vi "nana_4-solanka.vi"() -> ()   [LabVIEW 2015]
uses:
  <vilib>/MakerHub/LINX/Public/Peripherals/Digital/Digital Write N Chans.vi
  <vilib>/MakerHub/LINX/Public/Peripherals/Analog/Analog Read 1 Chan.vi
  <vilib>/MakerHub/LINX/Private/Local IO/LinxDigitalWrite.vi
  <vilib>/MakerHub/LINX/Public/Utilities/Check Channel.vi
  <vilib>/MakerHub/LINX/Public/Peripherals/Analog/Analog Read N Chans.vi
  <vilib>/MakerHub/LINX/Private/Local IO/LinxAnalogRead.vi
  <vilib>/MakerHub/LINX/Public/Utilities/Open Serial.vi
  <vilib>/MakerHub/LINX/Private/Utilties/Generate Error.vi
  <vilib>/MakerHub/LINX/LMH-LINX.lvlib
panel:
  in  "time post":u32
  in  "number of pulses":i32
  in  "low delay":u32
  in  "peak delay":u32
  out "Ref":dbl(graph)
  in  "LED":refnum<visa-resource-name>="N/A"
  out "3":dbl(graph)
  out "2":dbl(graph)
  out "4":dbl(graph)
  out "1":dbl(graph)
  out "pos":dbl
  in  "milliseconds to wait":u32
  in  "time pre":u32
  in  "Serial Port Analog":refnum<visa-resource-name>="N/A"
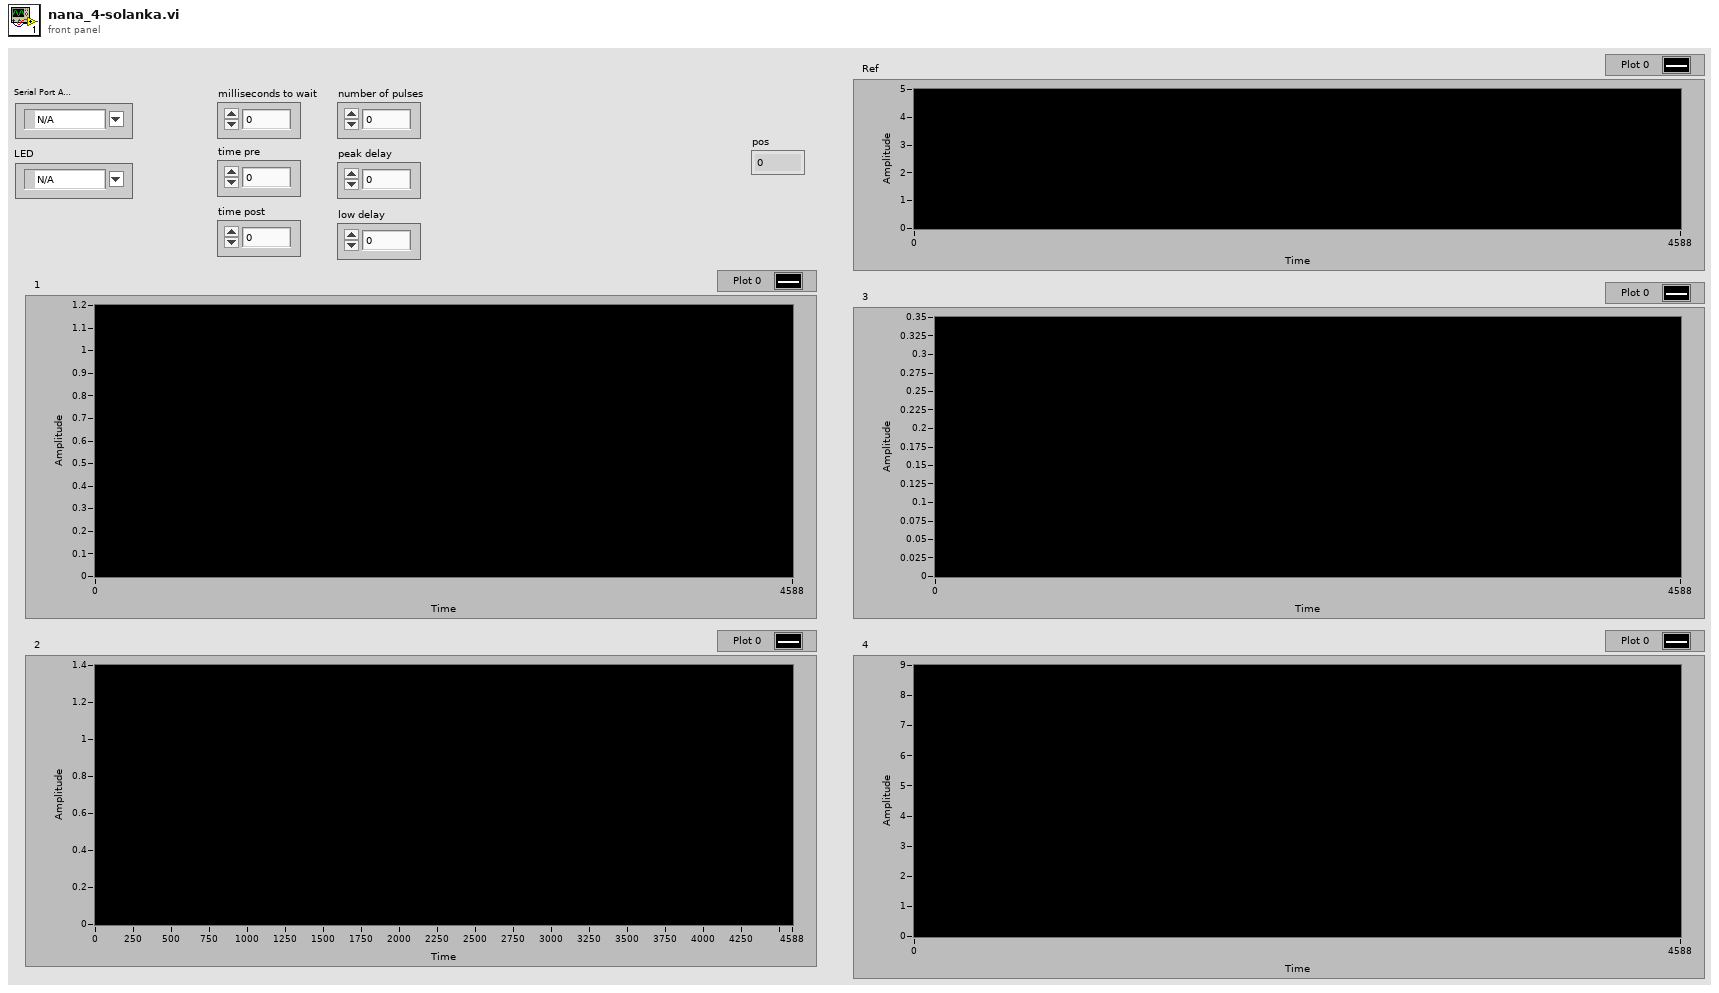
[diagram p1: front panel]
types:
  T1 = typedef "LMH-LINX.lvlib/LINX Ref.ctl" = cluster{"IO":T2, "Interface":T3, "LINX Device Config":T4}
  T2 = typedef "LMH-LINX.lvlib/Platform.ctl" = enum16{"Remote", "Local"}
  T3 = typedef "LMH-LINX.lvlib/Interface.ctl" = enum16{"Serial", "TCP"}
  T4 = typedef "LMH-LINX.lvlib/Device.lvlib/LINX Device Config.ctl" = cluster{"Interface":T3, "COM Port":refnum<visa-resource-name>, "TCP Configuration":T5, "Device Family":u8, "Device ID":u8, "Device Name":string, "TCP Ref":refnum<k5>, "Channels":T6}
  T5 = typedef "LMH-LINX.lvlib/Device.lvlib/TCP Config.ctl" = cluster{"IP Address":string, "Port":u16}
  T6 = typedef "LMH-LINX.lvlib/Channels.ctl" = cluster{"DI":u8[], "DO":u8[], "AI":u8[], "AO":u8[], "PWM":u8[], "QE":u8[], "UART":u8[], "I2C 2":u8[], "SPI":u8[], "CAN":u8[], "Servo":u8[], "AI Ref (V)":dbl, "AI Resolution (Bits)":u8, "AO Ref (V)":dbl, "AO Resolution (Bits)":u8}
  T7 = enum16{"open", "replace", "create", "open or create", "replace or create", "replace or create with confirmation"}
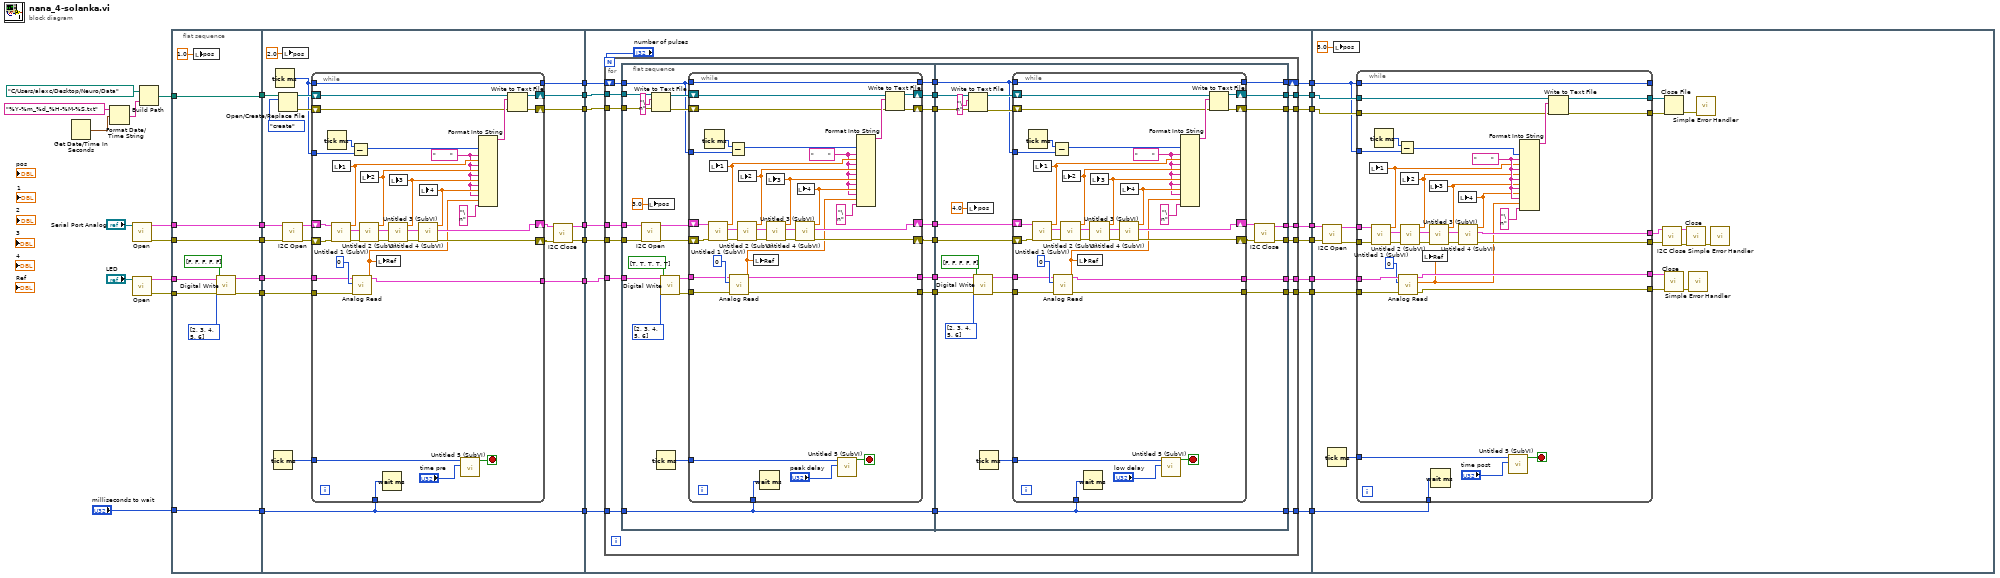
[diagram p0: block diagram]
diagram:
  n1 = Get Date/Time In Seconds() -> (seconds since 1Jan1904=w11:timestamp)
  n2 = Format Date/Time String(time format string (%c)="%Y-%m_%d_%H-%M-%S.txt", seconds (now)=w11) -> (date/time string=w13:string)  [unwired: 1 in]
  n3 = call-poly <vilib>:"Open.vi"("Serial Port"="Serial Port Analog") -> ("Error Out"=w17:errorcluster, "LINX Resource"=w18:T1)  [unwired: 8 in, 1 out]
  n4 = call-poly <vilib>:"Open.vi"("Serial Port"="LED") -> ("Error Out"=w8:errorcluster, "LINX Resource"=w9:T1)  [unwired: 8 in, 1 out]
  n5 = Build Path(base path=path "C:/Users/alexc/Desktop/Neuro/Data", name or relative path=w13) -> (appended path=w10:path)
  n6 = flat-sequence {
    tunnel: [w41] -> w33
    tunnel: [w40] -> w32
    tunnel: [w39] -> w29
    tunnel: [w34] -> w20
    tunnel: w18 -> [w41]
    tunnel: w17 -> [w40]
    tunnel: w10 -> [w39]
    tunnel: w9 -> [w38]
    tunnel: w8 -> [w37]
    tunnel: [w36] -> w7
    tunnel: [w35] -> w6
    tunnel: "milliseconds to wait" -> [w34]
    tunnel: w33 -> [w66]
    tunnel: w32 -> [w65]
    tunnel: [w64] -> w31
    tunnel: [w63] -> w30
    tunnel: w29 -> [w62]
    tunnel: [w58] -> w28
    tunnel: [w57] -> w27
    tunnel: [w55] -> w26
    tunnel: w20 -> [w53]
    tunnel: [w53] -> w19
    tunnel: w7 -> [w47]
    tunnel: w6 -> [w46]
    tunnel: [w45] -> w5
    tunnel: [w105] -> w25
    tunnel: [w104] -> w24
    tunnel: [w108] -> w23
    tunnel: [w107] -> w22
    tunnel: [w106] -> w21
    tunnel: w19 -> [w109]
    tunnel: w26 -> [w113]
    tunnel: w27 -> [w114]
    tunnel: w28 -> [w115]
    tunnel: w30 -> [w111]
    tunnel: w31 -> [w112]
    tunnel: w5 -> [w116]
    tunnel: [w103] -> w3
    tunnel: [w102] -> w2
    tunnel: [w101] -> w1
    tunnel: w21 -> [w274]
    tunnel: w22 -> [w275]
    tunnel: w23 -> [w261]
    tunnel: w24 -> [w279]
    tunnel: w25 -> [w283]
    tunnel: w3 -> [w278]
    tunnel: w2 -> [w265]
    tunnel: w1 -> [w264]
    frame #0 {
      n7 = local write "pos"(1.0 ("pos")) -> ()
      n8 = call-poly <vilib>:"Digital Write.vi"("Error In"=w37, "Values"=bool[] [FALSE, FALSE, FALSE, FALSE, FALSE], "DO Channels"=u8[] [2, 3, 4, 5, 6], "LINX Resource"=w38) -> ("Error Out"=w35:errorcluster, "LINX Resource"=w36:T1)  [unwired: 6 in]
    }
    frame #1 {
      n9 = Tick Count (ms)() -> (millisecond timer value=w54:u32)
      n10 = Tick Count (ms)() -> (millisecond timer value=w56:u32)
      n11 = Open/Create/Replace File(file path (use dialog)=w62, operation (0:open)=T7."create") -> (refnum out=w60:refnum<file>, error out=w59:errorcluster)  [unwired: 4 in, 1 out]
      n12 = local write "pos"(2.0 ("pos")) -> ()
      n13 = call <vilib>:"I2C Open.vi"("Error In"=w65, "LINX Resource"=w66) -> ("Error Out"=w51:errorcluster, "LINX Resource"=w52:T1)  [unwired: 8 in]
      n14 = while {
        tunnel: w56 -> [w93]
        shift-right: [w89] -> w58
        shift-left: w60 -> [w91]
        shift-right: [w88] -> w57
        shift-left: w59 -> [w90]
        tunnel: [w87] -> w55
        tunnel: w56 -> [w87]
        tunnel: w54 -> [w86]
        tunnel: w53 -> [w68]
        shift-right: [w83] -> w50
        shift-left: w52 -> [w85]
        shift-right: [w82] -> w49
        shift-left: w51 -> [w84]
        tunnel: w47 -> [w71]
        tunnel: w46 -> [w70]
        tunnel: [w67] -> w45
        stop <- w69 stop-if-true
        w75 = "       "
        n15 = Tick Count (ms)() -> (millisecond timer value=w94:u32)
        n16 = call "Untitled 1 (SubVI).vi"("error in (no error)"=w84, "LINX Resource in"=w85) -> ("error out"=w99:errorcluster, "LINX Resource out"=w100:T1, "Numeric"=w80:dbl)  [unwired: 7 in]
        n17 = local write "1"(w80) -> ()
        n18 = Subtract(x=w94, y=w93) -> (x-y=w76:u32)
        n19 = call-poly <vilib>:"Analog Read.vi"("Error In"=w70, "Analog Channel"=u8 0, "LINX Resource"=w71) -> ("Voltage"=w72:dbl, "LINX Resource"=w67:T1)  [unwired: 5 in, 2 out]
        n20 = call "Untitled 2 (SubVI).vi"("error in (no error)"=w99, "LINX Resource in"=w100) -> ("error out"=w98:errorcluster, "LINX Resource"=w97:T1, "Numeric"=w79:dbl)  [unwired: 7 in]
        n21 = local write "2"(w79) -> ()
        n22 = local write "Ref"(w72) -> ()
        n23 = Wait (ms)(milliseconds to wait=w68) -> ()  [unwired: 1 out]
        n24 = call "Untitled 3 (SubVI).vi"("error in (no error)"=w98, "LINX Resource in"=w97) -> ("error out"=w95:errorcluster, "LINX Resource out"=w96:T1, "Numeric"=w78:dbl)  [unwired: 7 in]
        n25 = local write "3"(w78) -> ()
        n26 = call "Untitled 4 (SubVI).vi"("error in (no error)"=w95, "LINX Resource in"=w96) -> ("error out"=w82:errorcluster, "LINX Resource"=w83:T1, "Numeric"=w81:dbl)  [unwired: 7 in]
        n27 = local write "4"(w81) -> ()
        n28 = call "Untitled 5 (SubVI).vi"("time_1"="time pre", "millisecond timer value"=w86) -> ("Boolean"=w69:bool)  [unwired: 9 in]
        n29 = Format Into String(w76, w75, w80, w75, w79, w75, w78, w75, w81, w75, w72, "\n") -> (resulting string=w92:string)  [unwired: 3 in, 1 out]
        n30 = Write to Text File(file (use dialog)=w91, text=w92, error in=w90) -> (refnum out=w89:refnum<file>, error out=w88:errorcluster)  [unwired: 1 in, 1 out]
      }
      n31 = call <vilib>:"I2C Close.vi"("Error In"=w49, "LINX Resource"=w50) -> ("Error Out"=w63:errorcluster, "LINX Resource"=w64:T1)  [unwired: 8 in]
    }
    frame #2 {
      n32 = for {
        N: "number of pulses" -> [_]
        tunnel: w116 -> [w139]
        tunnel: w115 -> [w138]
        tunnel: w114 -> [w137]
        shift-right: [w124] -> w108
        shift-left: w113 -> [w134]
        tunnel: w112 -> [w136]
        tunnel: w111 -> [w135]
        tunnel: w109 -> [w126]
        tunnel: [w123] -> w107
        tunnel: [w122] -> w106
        tunnel: [w121] -> w105
        tunnel: [w120] -> w104
        tunnel: [w119] -> w103
        tunnel: [w118] -> w102
        tunnel: [w117] -> w101
        n33 = flat-sequence {
          tunnel: w139 -> [w159]
          tunnel: w138 -> [w156]
          tunnel: w137 -> [w155]
          tunnel: w136 -> [w148]
          tunnel: w135 -> [w147]
          tunnel: w134 -> [w144]
          tunnel: [w163] -> w133
          tunnel: [w162] -> w132
          tunnel: [w158] -> w131
          tunnel: [w157] -> w130
          tunnel: [w152] -> w129
          tunnel: [w151] -> w128
          tunnel: [w143] -> w127
          tunnel: w126 -> [w140]
          tunnel: [w140] -> w125
          tunnel: w133 -> [w218]
          tunnel: w132 -> [w217]
          tunnel: w131 -> [w212]
          tunnel: w130 -> [w211]
          tunnel: w129 -> [w214]
          tunnel: w128 -> [w213]
          tunnel: w127 -> [w210]
          tunnel: w125 -> [w202]
          tunnel: [w207] -> w124
          tunnel: [w206] -> w123
          tunnel: [w205] -> w122
          tunnel: [w204] -> w121
          tunnel: [w203] -> w120
          tunnel: [w202] -> w119
          tunnel: [w201] -> w118
          tunnel: [w200] -> w117
          frame #0 {
            n34 = call <vilib>:"I2C Open.vi"("Error In"=w147, "LINX Resource"=w148) -> ("Error Out"=w145:errorcluster, "LINX Resource"=w146:T1)  [unwired: 8 in]
            n35 = local write "pos"(3.0 ("pos")) -> ()
            n36 = Write to Text File(file (use dialog)=w156, text="\n", error in=w155) -> (refnum out=w154:refnum<file>, error out=w153:errorcluster)  [unwired: 1 in, 1 out]
            n37 = Tick Count (ms)() -> (millisecond timer value=w141:u32)
            n38 = call-poly <vilib>:"Digital Write.vi"("Values"=bool[] [TRUE, TRUE, TRUE, TRUE, TRUE], "DO Channels"=u8[] [2, 3, 4, 5, 6], "LINX Resource"=w159) -> ("Error Out"=w150:errorcluster, "LINX Resource"=w149:T1)  [unwired: 7 in]
            n39 = while {
              tunnel: w144 -> [w192]
              shift-right: [w188] -> w158
              shift-left: w154 -> [w190]
              shift-right: [w187] -> w157
              shift-left: w153 -> [w189]
              tunnel: [w186] -> w143
              tunnel: w144 -> [w186]
              tunnel: w141 -> [w185]
              tunnel: w140 -> [w167]
              shift-right: [w182] -> w163
              shift-left: w146 -> [w184]
              shift-right: [w181] -> w162
              shift-left: w145 -> [w183]
              tunnel: w149 -> [w170]
              tunnel: w150 -> [w169]
              tunnel: [w166] -> w152
              tunnel: [w165] -> w151
              stop <- w168 stop-if-true
              w174 = "       "
              n40 = Tick Count (ms)() -> (millisecond timer value=w193:u32)
              n41 = call "Untitled 1 (SubVI).vi"("error in (no error)"=w183, "LINX Resource in"=w184) -> ("error out"=w198:errorcluster, "LINX Resource out"=w199:T1, "Numeric"=w179:dbl)  [unwired: 7 in]
              n42 = local write "1"(w179) -> ()
              n43 = Subtract(x=w193, y=w192) -> (x-y=w175:u32)
              n44 = call-poly <vilib>:"Analog Read.vi"("Error In"=w169, "Analog Channel"=u8 0, "LINX Resource"=w170) -> ("Error Out"=w165:errorcluster, "Voltage"=w171:dbl, "LINX Resource"=w166:T1)  [unwired: 5 in, 1 out]
              n45 = call "Untitled 2 (SubVI).vi"("error in (no error)"=w198, "LINX Resource in"=w199) -> ("error out"=w197:errorcluster, "LINX Resource"=w196:T1, "Numeric"=w178:dbl)  [unwired: 7 in]
              n46 = local write "2"(w178) -> ()
              n47 = local write "Ref"(w171) -> ()
              n48 = Wait (ms)(milliseconds to wait=w167) -> ()  [unwired: 1 out]
              n49 = call "Untitled 3 (SubVI).vi"("error in (no error)"=w197, "LINX Resource in"=w196) -> ("error out"=w194:errorcluster, "LINX Resource out"=w195:T1, "Numeric"=w177:dbl)  [unwired: 7 in]
              n50 = local write "3"(w177) -> ()
              n51 = call "Untitled 4 (SubVI).vi"("error in (no error)"=w194, "LINX Resource in"=w195) -> ("error out"=w181:errorcluster, "LINX Resource"=w182:T1, "Numeric"=w180:dbl)  [unwired: 7 in]
              n52 = local write "4"(w180) -> ()
              n53 = call "Untitled 5 (SubVI).vi"("time_1"="peak delay", "millisecond timer value"=w185) -> ("Boolean"=w168:bool)  [unwired: 9 in]
              n54 = Format Into String(w175, w174, w179, w174, w178, w174, w177, w174, w180, w174, w171, "\n") -> (resulting string=w191:string)  [unwired: 3 in, 1 out]
              n55 = Write to Text File(file (use dialog)=w190, text=w191, error in=w189) -> (refnum out=w188:refnum<file>, error out=w187:errorcluster)  [unwired: 1 in, 1 out]
            }
          }
          frame #1 {
            n56 = local write "pos"(4.0 ("pos")) -> ()
            n57 = Write to Text File(file (use dialog)=w212, text="\n", error in=w211) -> (refnum out=w220:refnum<file>, error out=w221:errorcluster)  [unwired: 1 in, 1 out]
            n58 = call-poly <vilib>:"Digital Write.vi"("Error In"=w213, "Values"=bool[] [FALSE, FALSE, FALSE, FALSE, FALSE], "DO Channels"=u8[] [2, 3, 4, 5, 6], "LINX Resource"=w214) -> ("Error Out"=w225:errorcluster, "LINX Resource"=w224:T1)  [unwired: 6 in]
            n59 = Tick Count (ms)() -> (millisecond timer value=w208:u32)
            n60 = while {
              tunnel: w210 -> [w253]
              shift-right: [w249] -> w206
              shift-left: w220 -> [w251]
              shift-right: [w248] -> w205
              shift-left: w221 -> [w250]
              tunnel: [w247] -> w207
              tunnel: w210 -> [w247]
              tunnel: w208 -> [w246]
              tunnel: w202 -> [w228]
              shift-right: [w243] -> w216
              shift-left: w218 -> [w245]
              shift-right: [w242] -> w215
              shift-left: w217 -> [w244]
              tunnel: w224 -> [w231]
              tunnel: w225 -> [w230]
              tunnel: [w227] -> w201
              tunnel: [w226] -> w200
              stop <- w229 stop-if-true
              w235 = "       "
              n61 = Tick Count (ms)() -> (millisecond timer value=w254:u32)
              n62 = call "Untitled 1 (SubVI).vi"("error in (no error)"=w244, "LINX Resource in"=w245) -> ("error out"=w259:errorcluster, "LINX Resource out"=w260:T1, "Numeric"=w240:dbl)  [unwired: 7 in]
              n63 = local write "1"(w240) -> ()
              n64 = Subtract(x=w254, y=w253) -> (x-y=w236:u32)
              n65 = call-poly <vilib>:"Analog Read.vi"("Error In"=w230, "Analog Channel"=u8 0, "LINX Resource"=w231) -> ("Error Out"=w226:errorcluster, "Voltage"=w232:dbl, "LINX Resource"=w227:T1)  [unwired: 5 in, 1 out]
              n66 = call "Untitled 2 (SubVI).vi"("error in (no error)"=w259, "LINX Resource in"=w260) -> ("error out"=w258:errorcluster, "LINX Resource"=w257:T1, "Numeric"=w239:dbl)  [unwired: 7 in]
              n67 = local write "2"(w239) -> ()
              n68 = local write "Ref"(w232) -> ()
              n69 = Wait (ms)(milliseconds to wait=w228) -> ()  [unwired: 1 out]
              n70 = call "Untitled 3 (SubVI).vi"("error in (no error)"=w258, "LINX Resource in"=w257) -> ("error out"=w255:errorcluster, "LINX Resource out"=w256:T1, "Numeric"=w238:dbl)  [unwired: 7 in]
              n71 = local write "3"(w238) -> ()
              n72 = call "Untitled 4 (SubVI).vi"("error in (no error)"=w255, "LINX Resource in"=w256) -> ("error out"=w242:errorcluster, "LINX Resource"=w243:T1, "Numeric"=w241:dbl)  [unwired: 7 in]
              n73 = local write "4"(w241) -> ()
              n74 = call "Untitled 5 (SubVI).vi"("time_1"="low delay", "millisecond timer value"=w246) -> ("Boolean"=w229:bool)  [unwired: 9 in]
              n75 = Format Into String(w236, w235, w240, w235, w239, w235, w238, w235, w241, w235, w232, "\n") -> (resulting string=w252:string)  [unwired: 3 in, 1 out]
              n76 = Write to Text File(file (use dialog)=w251, text=w252, error in=w250) -> (refnum out=w249:refnum<file>, error out=w248:errorcluster)  [unwired: 1 in, 1 out]
            }
            n77 = call <vilib>:"I2C Close.vi"("Error In"=w215, "LINX Resource"=w216) -> ("Error Out"=w203:errorcluster, "LINX Resource"=w204:T1)  [unwired: 8 in]
          }
        }
      }
    }
    frame #3 {
      n78 = call <vilib>:"I2C Open.vi"("Error In"=w279, "LINX Resource"=w283) -> ("Error Out"=w276:errorcluster, "LINX Resource"=w277:T1)  [unwired: 8 in]
      n79 = Tick Count (ms)() -> (millisecond timer value=w273:u32)
      n80 = local write "pos"(5.0 ("pos")) -> ()
      n81 = while {
        tunnel: w278 -> [w310]
        tunnel: w277 -> [w309]
        tunnel: w276 -> [w308]
        tunnel: [w302] -> _
        tunnel: w261 -> [w302]
        tunnel: w275 -> [w301]
        tunnel: w274 -> [w300]
        tunnel: w273 -> [w299]
        tunnel: [w298] -> w272
        tunnel: [w297] -> w271
        tunnel: [w296] -> w268
        tunnel: [w295] -> w267
        tunnel: w265 -> [w294]
        tunnel: w264 -> [w293]
        tunnel: [w292] -> w263
        tunnel: [w291] -> w262
        tunnel: w261 -> [w289]
        stop <- w311 stop-if-true
        w314 = "       "
        n82 = call "Untitled 1 (SubVI).vi"("error in (no error)"=w308, "LINX Resource in"=w309) -> ("error out"=w307:errorcluster, "LINX Resource out"=w318:T1, "Numeric"=w304:dbl)  [unwired: 7 in]
        n83 = local write "1"(w304) -> ()
        n84 = Tick Count (ms)() -> (millisecond timer value=w303:u32)
        n85 = Subtract(x=w303, y=w289) -> (x-y=w288:u32)
        n86 = call-poly <vilib>:"Analog Read.vi"("Error In"=w293, "Analog Channel"=u8 0, "LINX Resource"=w294) -> ("Error Out"=w291:errorcluster, "Voltage"=w287:dbl, "LINX Resource"=w292:T1)  [unwired: 5 in, 1 out]
        n87 = call "Untitled 2 (SubVI).vi"("error in (no error)"=w307, "LINX Resource in"=w318) -> ("error out"=w306:errorcluster, "LINX Resource"=w317:T1, "Numeric"=w286:dbl)  [unwired: 7 in]
        n88 = local write "2"(w286) -> ()
        n89 = local write "Ref"(w287) -> ()
        n90 = call "Untitled 3 (SubVI).vi"("error in (no error)"=w306, "LINX Resource in"=w317) -> ("error out"=w305:errorcluster, "LINX Resource out"=w316:T1, "Numeric"=w285:dbl)  [unwired: 7 in]
        n91 = local write "3"(w285) -> ()
        n92 = Wait (ms)(milliseconds to wait=w310) -> ()  [unwired: 1 out]
        n93 = call "Untitled 4 (SubVI).vi"("error in (no error)"=w305, "LINX Resource in"=w316) -> ("error out"=w295:errorcluster, "LINX Resource"=w296:T1, "Numeric"=w284:dbl)  [unwired: 7 in]
        n94 = local write "4"(w284) -> ()
        n95 = call "Untitled 5 (SubVI).vi"("time_1"="time post", "millisecond timer value"=w299) -> ("Boolean"=w311:bool)  [unwired: 9 in]
        n96 = Format Into String(w288, w314, w304, w314, w286, w314, w285, w314, w284, w314, w287, "\n") -> (resulting string=w315:string)  [unwired: 3 in, 1 out]
        n97 = Write to Text File(file (use dialog)=w301, text=w315, error in=w300) -> (refnum out=w298:refnum<file>, error out=w297:errorcluster)  [unwired: 1 in, 1 out]
      }
      n98 = call <vilib>:"I2C Close.vi"("Error In"=w267, "LINX Resource"=w268) -> ("Error Out"=w269:errorcluster, "LINX Resource"=w270:T1)  [unwired: 8 in]
      n99 = Close File(refnum=w272, error in=w271) -> (error out=w282:errorcluster)  [unwired: 1 out]
      n100 = call <vilib>:"Close.vi"("Error In"=w262, "LINX Resource"=w263) -> ("Error Out"=w266:errorcluster)  [unwired: 9 in]
      n101 = call <vilib>:"Close.vi"("Error In"=w269, "LINX Resource"=w270) -> ("Error Out"=w281:errorcluster)  [unwired: 9 in]
      n102 = call <vilib>:"Simple Error Handler.vi"("error in (no error)"=w266) -> ()  [unwired: 4 in, 5 out]
      n103 = call <vilib>:"Simple Error Handler.vi"("error in (no error)"=w282) -> ()  [unwired: 4 in, 5 out]
      n104 = call <vilib>:"Simple Error Handler.vi"("error in (no error)"=w281) -> ()  [unwired: 4 in, 5 out]
    }
  }
